vi "parse websocket length header.vi"(11 "header string":string) -> (2 "mask(1)+length(7)":u8, 3 "first byte":T1 {"opcode" format="%.0x"})   [LabVIEW 2016, in "websocket core.lvlib"]
uses:
  websocket core.lvlib
  first byte header.ctl
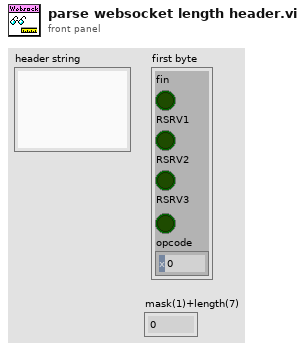
[diagram p1: front panel]
types:
  T1 = typedef "websocket core.lvlib/first byte header.ctl" = cluster{"fin":bool, "RSRV1":bool, "RSRV2":bool, "RSRV3":bool, "opcode":u8}
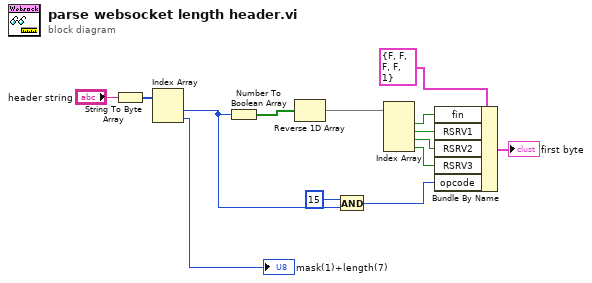
[diagram p0: block diagram]
diagram:
  n1 = String To Byte Array(string="header string") -> (unsigned byte array=w6:u8[])
  n2 = Index Array(array=w6) -> (element #1=w3:u8, element #2=→"mask(1)+length(7)":u8)  [unwired: 2 in]
  n3 = Number To Boolean Array(number=w3) -> (Boolean array=w8:bool[])
  n4 = Reverse 1D Array(array=w8) -> (reversed array=w4:bool[])
  n5 = And(x=u8 15, y=w3) -> (x .and. y?=w1:u8)
  n6 = Index Array(array=w4) -> (element #1=w10:bool, element #2=w13:bool, element #3=w12:bool, element #4=w11:bool)  [unwired: 4 in]
  n7 = Bundle By Name(cluster=T1 {"fin"=FALSE, "RSRV1"=FALSE, "RSRV2"=FALSE, "RSRV3"=FALSE, "opcode"=1} ("first byte"), "fin"=w10, "RSRV1"=w13, "RSRV2"=w12, "RSRV3"=w11, "opcode"=w1) -> (→"first byte":T1)
